vi "Measurement Logic.vi"() -> ()   [LabVIEW 2020, in "NIDigitalSPI.lvlib"]
uses:
  NIDigitalSPI.lvlib
  <instrlib>/niDigital/niDigital.llb/niDigital Load Specifications Levels and Timing (Single).vi
  <instrlib>/niDigital/niDigital.llb/niDigital Selected Function.ctl
  Measurement Results.ctl
  <instrlib>/niDigital/niDigital.llb/niDigital Burst Pattern (Pass Fail).vi
  <vilib>/MeasurementLink/MeasurementLink niDigital/MeasurementLink niDigital.lvlib
  <vilib>/MeasurementLink/MeasurementLink niDigital/Initialize Sessions - 1Sess.vi
  <vilib>/MeasurementLink/MeasurementLink Measurement Server/Measure Call Context/Measure Call Context.lvclass
  <vilib>/MeasurementLink/MeasurementLink Session Management V1/Session Reservation/Session Reservation.lvclass
  Measurement Configuration.ctl
panel:
  out "measure call context out":refnum<class "Measure Call Context.lvclass">
  in  "measure call context in":refnum<class "Measure Call Context.lvclass">
  out "measurement results":T1
  in  "measurement configuration":T2
  out "error out":errorcluster
  in  "error in":errorcluster
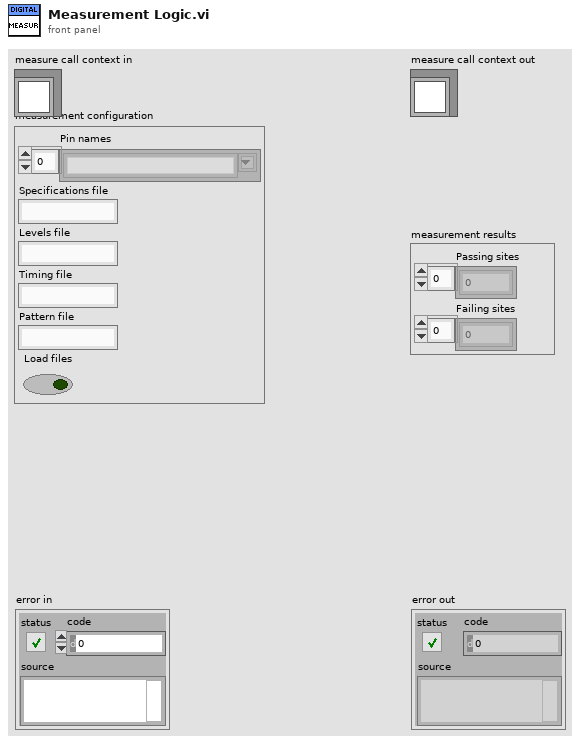
[diagram p1: front panel]
types:
  T1 = typedef "NIDigitalSPI.lvlib/Measurement Results.ctl" = cluster{"Passing sites":i32[], "Failing sites":i32[]}
  T2 = typedef "NIDigitalSPI.lvlib/Measurement Configuration.ctl" = cluster{"Pin names":string[], "Specifications file":string, "Levels file":string, "Timing file":string, "Pattern file":string, "Load files":bool}
  T3 = typedef "niDigital Selected Function.ctl" = i32
  T4 = typedef "MeasurementLink Measurement Server.lvlib/PinMapContext.ctl" = cluster{"pin_map_id":string, "sites":i32[]}
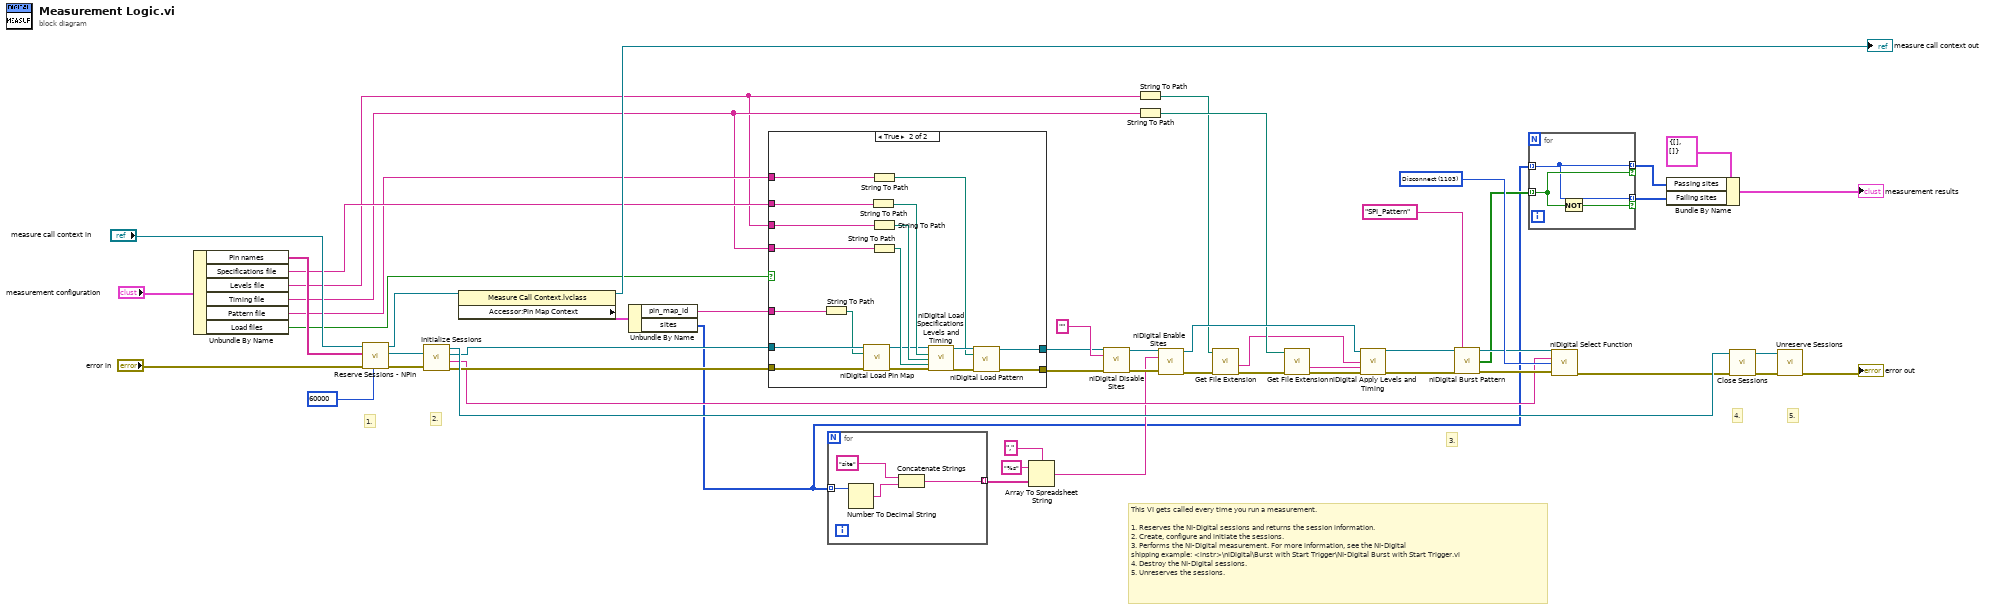
[diagram p0: block diagram]
diagram:
  w31 = T3 1103 items=["Digital"=1100, "PPMU"=1101, "Off"=1102, "Disconnect"=1103] ("function")
  # "This VI gets called every time you run a measurement.\n\n1. Reserves the NI-Digital sessions and returns the session information.\n2. Create, configure and initiate the sessions.\n3. Performs the NI-Digital measurement. For more information, see the NI-Digital\nshipping example: <instr>\\niDigital\\Burst with Start Trigger\\NI-Digital Burst with Start Trigger.vi\n4. Destroy the NI-Digital sessions.\n5. Unreserves the sessions."
  # "5."
  # "4."
  # "3."
  # "2."
  # "1."
  n1 = Unbundle By Name("measurement configuration") -> ("Pin names"=w48:string[], "Specifications file"=w36:string, "Levels file"=w5:string, "Timing file"=w8:string, "Pattern file"=w35:string, "Load files"=w21:bool)
  n2 = call <vilib>:"Reserve Sessions - NPin.vi"("timeout (ms)"=60000 ("timeout in milliseconds"), "error in"="error in", "pin or relay names"=w48, "measurement context in"="measure call context in") -> ("error out"=w45:errorcluster, "session reservation out"=w44:refnum<class "Session Reservation.lvclass">, "measurement context out"=w46:refnum<class "Measure Call Context.lvclass">)  [unwired: 5 in]
  n3 = call-poly <vilib>:"Initialize Sessions.vi"("error in"=w45, "session reservation in"=w44) -> ("error out"=w39:errorcluster, "channel list"=w29:string, "session"=w38:refnum<k15>, "session reservation out"=w40:refnum<class "Session Reservation.lvclass">)  [unwired: 6 in]
  n4 = property class="Measure Call Context.lvclass"(reference=w46) -> (reference out=→"measure call context out":refnum<class "Measure Call Context.lvclass">, "Accessor:Pin Map Context"=w52:T4)  [unwired: 1 in, 1 out]
  n5 = Unbundle By Name(w52) -> ("pin_map_id"=w37:string, "sites"=w10:i32[])
  n6 = case shown="True" w21 {
    tunnel: w39 -> [w54 w73]
    tunnel: w38 -> [w55 w72]
    tunnel: w37 -> [_ w71]
    tunnel: w36 -> [_ w68]
    tunnel: w35 -> [_ w61]
    tunnel: [w54 w59] -> w19
    tunnel: [w55 w58] -> w18
    tunnel: w5 -> [_ w57]
    tunnel: w8 -> [_ w56]
    frame False {
      # "When running this measurement from TestStand, TestStand should have already loaded the pin map, specifications, levels, timing, and pattern so there is no need to load those files again."
    }
    frame True {
      n7 = String To Path(string=w71) -> (path=w70:path)
      n8 = call <instrlib>:"niDigital Load Pin Map.vi"("instrument handle"=w72, "pin map file"=w70, "error in"=w73) -> ("instrument handle out"=w64:refnum<k15>, "error out"=w69:errorcluster)  [unwired: 11 in]
      n9 = String To Path(string=w68) -> (path=w65:path)
      n10 = String To Path(string=w61) -> (path=w60:path)
      n11 = String To Path(string=w57) -> (path=w66:path)
      n12 = String To Path(string=w56) -> (path=w67:path)
      n13 = call-poly <instrlib>:"niDigital Load Specifications Levels and Timing.vi"("instrument handle"=w64, "specifications file path"=w65, "levels file path"=w66, "timing file path"=w67, "error in"=w69) -> ("instrument handle out"=w62:refnum<k15>, "error out"=w63:errorcluster)  [unwired: 9 in]
      n14 = call <instrlib>:"niDigital Load Pattern.vi"("instrument handle"=w62, "pattern file"=w60, "error in"=w63) -> ("instrument handle out"=w58:refnum<k15>, "error out"=w59:errorcluster)  [unwired: 11 in]
    }
  }
  n15 = for {
    tunnel: w10 -> [w76] mode=indexing
    tunnel: [w74] -> w14 mode=indexing
    n16 = Number To Decimal String(number=w76) -> (decimal integer string=w75:string)  [unwired: 1 in]
    n17 = Concatenate Strings("site" ("string"), w75) -> (w74:string)
  }
  n18 = Array To Spreadsheet String(delimiter (Tab)=",", array=w14, 3:"%s" ("format string")) -> (spreadsheet string=w11:string)
  n19 = call <instrlib>:"niDigital Disable Sites.vi"("instrument handle"=w18, "site list"="", "error in"=w19) -> ("instrument handle out"=w16:refnum<k15>, "error out"=w17:errorcluster)  [unwired: 11 in]
  n20 = String To Path(string=w5) -> (path=w6:path)
  n21 = String To Path(string=w8) -> (path=w9:path)
  n22 = call <instrlib>:"niDigital Enable Sites.vi"("instrument handle"=w16, "site list"=w11, "error in"=w17) -> ("instrument handle out"=w15:refnum<k15>, "error out"=w1:errorcluster)  [unwired: 11 in]
  n23 = call <vilib>:"Get File Extension.vi"("error in (no error)"=w1, "file"=w6) -> ("error out"=w3:errorcluster, "filename without extension"=w4:string)  [unwired: 5 in, 3 out]
  n24 = call <vilib>:"Get File Extension.vi"("error in (no error)"=w3, "file"=w9) -> ("error out"=w2:errorcluster, "filename without extension"=w7:string)  [unwired: 5 in, 3 out]
  n25 = call <instrlib>:"niDigital Apply Levels and Timing.vi"("instrument handle"=w15, "levels sheet"=w4, "timing sheet"=w7, "error in"=w2) -> ("instrument handle out"=w33:refnum<k15>, "error out"=w34:errorcluster)  [unwired: 10 in]
  n26 = call-poly <instrlib>:"niDigital Burst Pattern.vi"("instrument handle"=w33, "start label"="SPI_Pattern", "error in"=w34) -> ("instrument handle out"=w27:refnum<k15>, "pass"=w23:bool[], "error out"=w30:errorcluster)  [unwired: 10 in]
  n27 = for {
    tunnel: w23 -> [w80] mode=indexing
    tunnel: [w78] -> w25 mode=indexing if=w80
    tunnel: [w78] -> w24 mode=indexing if=w79
    tunnel: w10 -> [w78] mode=indexing
    n28 = Not(x=w80) -> (.not. x?=w79:bool)
  }
  n29 = call <instrlib>:"niDigital Select Function.vi"("instrument handle"=w27, "channel list"=w29, "function"=w31, "error in"=w30) -> ("error out"=w28:errorcluster)  [unwired: 10 in, 1 out]
  n30 = Bundle By Name(cluster=T1 {"Passing sites"=[], "Failing sites"=[]} ("Measurement Results"), "Passing sites"=w25, "Failing sites"=w24) -> (→"measurement results":T1)
  n31 = call <vilib>:"Close Sessions.vi"("error in"=w28, "session reservation in"=w40) -> ("error out"=w42:errorcluster, "session reservation out"=w41:refnum<class "Session Reservation.lvclass">)  [unwired: 8 in]
  n32 = call <vilib>:"Unreserve Sessions.vi"("error in"=w42, "session reservation in"=w41) -> ("error out"=→"error out":errorcluster)  [unwired: 9 in]
